vi "Get Compare List.vi"(8 "error in (no error)":errorcluster, 11 "I2C waveform info":T2) -> (0 "error out":errorcluster, 1 "Compare types":T1[](array[typedef]), 2 "Compare locations":u64[](array[numeric]), 3 "I2C waveform info out":T2)   [LabVIEW 2009, in "IDW.lvlib"]
uses:
  IDW.lvlib
  _Typedefs/Waveform info.ctl
  _Typedefs/Timing - ticks.ctl
  _Typedefs/Default transition action.ctl
  _Typedefs/Bit type.ctl
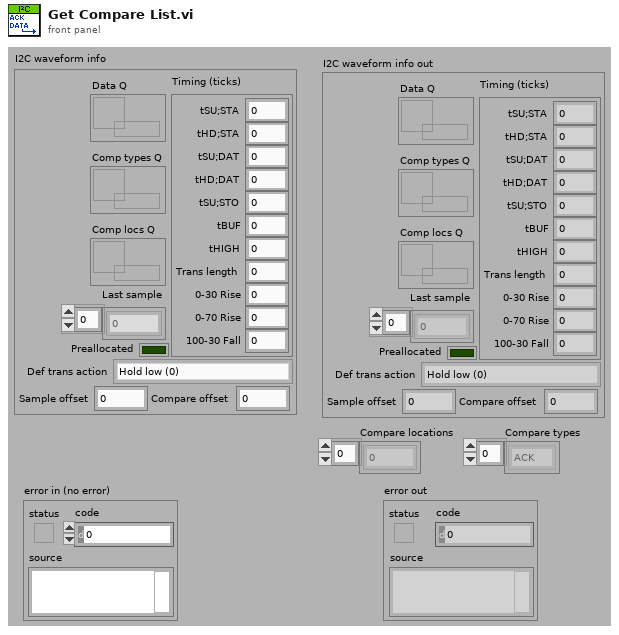
[diagram p1: front panel]
types:
  T1 = typedef "IDW.lvlib/Bit type.ctl" = enum16{"ACK", "Data"}
  T2 = typedef "IDW.lvlib/Waveform info.ctl" = cluster{"Last sample":u8[], "Sample offset":u64, "Compare offset":u64, "Timing (ticks)":T3, "Preallocated":bool, "Def trans action":T4, "Data Q":refnum<queue>, "Comp types Q":refnum<queue>, "Comp locs Q":refnum<queue>}
  T3 = typedef "IDW.lvlib/Timing - ticks.ctl" = cluster{"tSU;STA":i32, "tHD;STA":i32, "tSU;DAT":i32, "tHD;DAT":i32, "tSU;STO":i32, "tBUF":i32, "tHIGH":i32, "Trans length":i32, "0-30 Rise":i32, "0-70 Rise":i32, "100-30 Fall":i32}
  T4 = typedef "IDW.lvlib/Default transition action.ctl" = enum16{"Hold low (0)", "Release (Z)", "Set up next value", "Hold previous value", "Preserve tHD;DAT and tSU;DAT"}
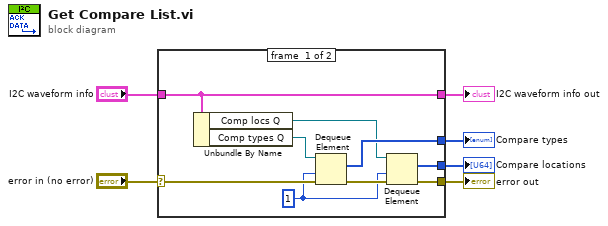
[diagram p0: block diagram]
diagram:
  n1 = case shown="No Error" "error in (no error)" {
    selector: "error in (no error)" -> [w13 w17]
    tunnel: [w15 w16] -> w3
    tunnel: "I2C waveform info" -> [w15 w16]
    tunnel: [w9 w17] -> w5
    tunnel: [w8 _] -> w2
    tunnel: [w12 _] -> w1
    frame #0 {
      w7 = 1 ("timeout in ms (-1)")
      n2 = Unbundle By Name(w15) -> ("Comp locs Q"=w11:refnum<queue>, "Comp types Q"=w14:refnum<queue>)
      n3 = Dequeue Element(queue=w14, timeout in ms (-1)=w7, error in (no error)=w13) -> (element=w12:T1[], error out=w10:errorcluster)  [unwired: 2 out]
      n4 = Dequeue Element(queue=w11, timeout in ms (-1)=w7, error in (no error)=w10) -> (element=w8:u64[], error out=w9:errorcluster)  [unwired: 2 out]
    }
    frame #1 {
    }
  }
  "error out" <- w5
  "I2C waveform info out" <- w3
  "Compare locations" <- w2
  "Compare types" <- w1
